vi "fgv_lookahead-pt.vi"(7 "cmd":enum16{"write", "read"}(ring), 11 "center":cluster{"x":dbl, "y":dbl}={"x"=175278.2659126866, "y"=530134.4315112913} {"x" format="%.2f"; "y" format="%.2f"}) -> (3 "loopahead-pt":cluster{"x":dbl, "y":dbl})   [LabVIEW 2019]
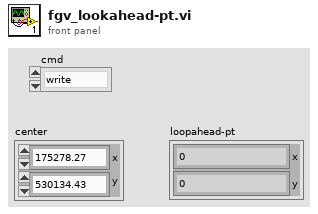
[diagram p1: front panel]
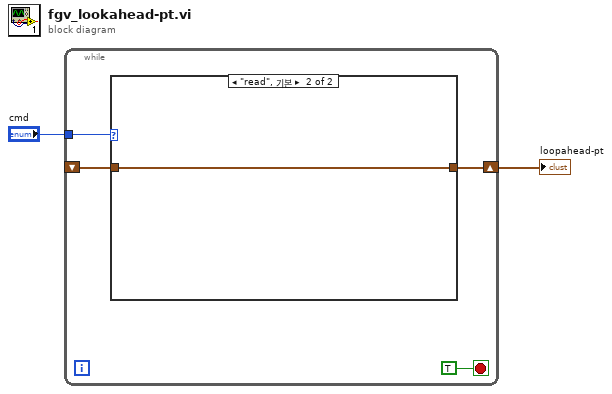
[diagram p0: block diagram]
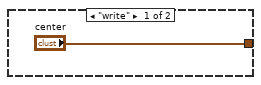
[diagram p2: hidden frame]
diagram:
  n1 = while {
    tunnel: "cmd" -> [w5]
    shift-right: [w4] -> w1
    shift-left: _ -> [w3]
    stop <- TRUE stop-if-true
    n2 = case shown="\"read\", 기본" w5 {
      tunnel: ["center" w8] -> w4
      tunnel: w3 -> [_ w8]
      frame "write" {
      }
      frame "read", Default {
      }
    }
  }
  "loopahead-pt" <- w1
